vi "Look In Map.vi"(0 "DBMap in":refnum<class "DBMap.lvclass">, 5 "Key":string, 11 "error in (no error)":errorcluster {"code" format="Error %.0f"}) -> (4 "DBMap out":refnum<class "DBMap.lvclass">, 6 "File Data":T1, 8 "Not Found?":bool, 15 "error out":errorcluster {"code" format="Error %.0f"})   [LabVIEW 2024, in "DBMap.lvclass"]
uses:
  DBMap.lvclass
  DBMap.lvclass/DBMap.ctl
  <vilib>/drjdpowell/SQLite Library/SQLite.lvlib
  <vilib>/drjdpowell/SQLite Library/SQL Connection/Execute SQL (1D String).vi
  <vilib>/drjdpowell/SQLite Library/SQL Connection/Connection.lvclass
  File Metadata.ctl
  Node.ctl
  Source to Sink Array.ctl
  File Data.ctl
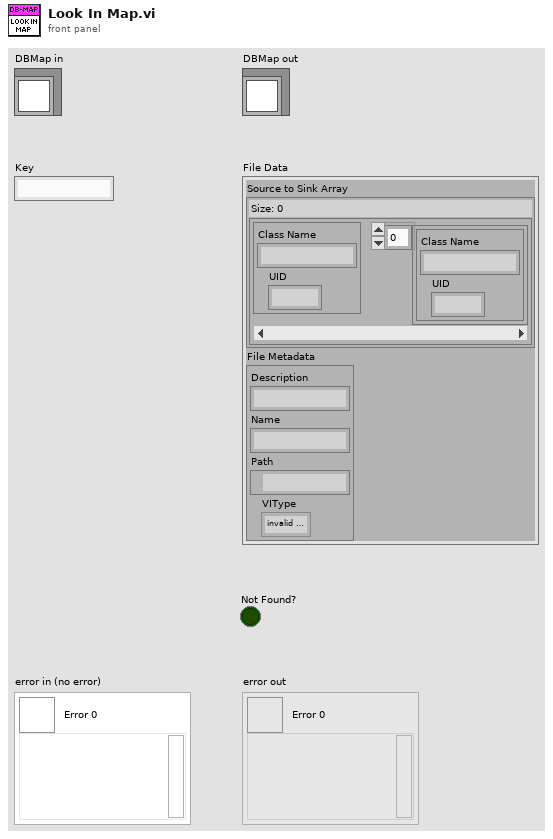
[diagram p1: front panel]
types:
  T1 = typedef "File Data.ctl" = cluster{"Source to Sink Array":T2, "File Metadata":T4}
  T2 = typedef "Source to Sink Array.ctl" = map{T3, T3[]}
  T3 = typedef "Node.ctl" = cluster{"Class Name":string, "UID":i32}
  T4 = typedef "File Metadata.ctl" = cluster{"Description":string, "Name":string, "Path":path, "VIType":enum32{"invalid VI type", "Standard VI", "Control VI", "Global VI", "Polymorphic VI", "Configuration VI", "SubSystem", "Facade VI", "Method VI", "Statechart Diagram VI"}}
  T5 = typedef "Semaphore RefNum" = refnum<k1>
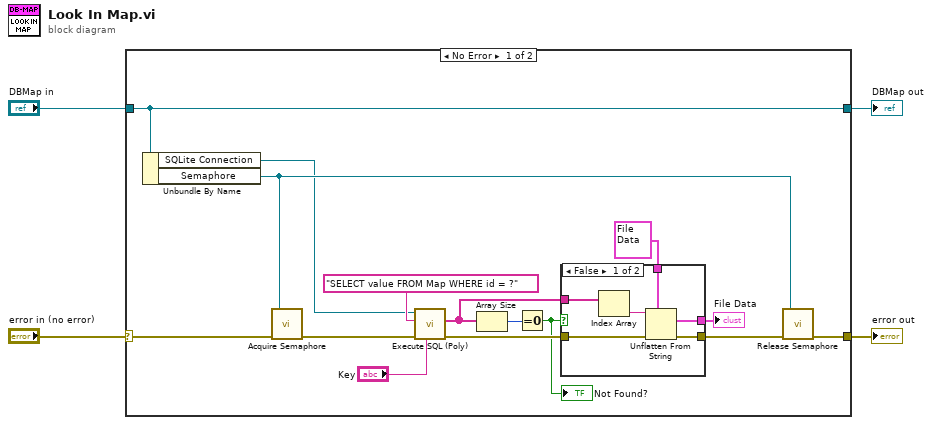
[diagram p0: block diagram]
diagram:
  n1 = case shown="No Error" "error in (no error)" {
    selector: "error in (no error)" -> [w18 w28]
    tunnel: [w17 w28] -> w3
    tunnel: [w19 w27] -> w1
    tunnel: "DBMap in" -> [w19 w27]
    frame No Error {
      n2 = Unbundle By Name(w19) -> ("SQLite Connection"=w7:refnum<class "Connection.lvclass">, "Semaphore"=w16:T5)
      n3 = call <vilib>:"Acquire Semaphore.vi"("error in (no error)"=w18, "semaphore"=w16) -> ("error out"=w8:errorcluster)  [unwired: 3 in, 2 out]
      n4 = call-poly <vilib>:"Execute SQL (Poly).vi"("Parameter(s)"="Key", "error in (no error)"=w8, "SQL"="SELECT value FROM Map WHERE id = ?", "SQLite Connection in"=w7) -> ("error out"=w14:errorcluster, "Result Set"=w12:string[])  [unwired: 4 in, 2 out]
      n5 = Array Size(array=w12) -> (size(s)=w11:i32)
      n6 = Equal To 0?(x=w11) -> (x = 0?=w10:bool)
      "Not Found?" <- w10
      n7 = case shown="False" w10 {
        tunnel: w14 -> [w25 w26]
        tunnel: [w24 w26] -> w9
        tunnel: w12 -> [w20 _]
        tunnel: T1 {"Source to Sink Array"={}, "File Metadata"={"Description"="", "Name"="", "Path"=path "", "VIType"=enum."invalid VI type"}} ("File Data") -> [w23 _]
        tunnel: [w22 _] -> w5
        frame False {
          n8 = Index Array(array=w20) -> (element=w21:string)  [unwired: 1 in]
          n9 = Unflatten From String(type=w23, binary string=w21, error in (no error)=w25) -> (value=w22:T1, error out=w24:errorcluster)  [unwired: 2 in, 1 out]
        }
        frame True {
        }
      }
      "File Data" <- w5
      n10 = call <vilib>:"Release Semaphore.vi"("error in (no error)"=w9, "semaphore"=w16) -> ("error out"=w17:errorcluster)  [unwired: 4 in, 1 out]
    }
    frame Error {
    }
  }
  "error out" <- w3
  "DBMap out" <- w1
